vi "MCLB Test.vi"() -> ()   [LabVIEW 2013]
uses:
  <vilib>/NI/Tag Bus/tag/Data Type.ctl
  Table Manager/object ref.ctl
  <vilib>/NI/Tag Bus Data Framework/Configuration Editor/Classes/Engine Parent/Engine Parent Editor Node.lvclass
  <vilib>/NI/Tag Bus Data Framework/Configuration Editor/Classes/Module editor node/module editor node.lvclass
  Table Manager/references.ctl
  <vilib>/NI/Configuration Framework/Node/StopEvent.ctl
  <vilib>/NI/Configuration Framework/Node/RefreshUIEvent.ctl
  <vilib>/NI/Configuration Framework/Node/CacheState.ctl
  <vilib>/NI/Configuration Framework/Node/NodeChangeEvent.ctl
  <vilib>/NI/Configuration Framework/Node/NodeRef.ctl
  <vilib>/NI/Configuration Framework/Node/NISE_CEF_Node.lvclass
  <vilib>/NI/Tag Bus Data Framework/control module/editor node/channel action event.ctl
  <vilib>/NI/Tag Bus Data Framework/control module/editor node/dialog output action.ctl
  <vilib>/NI/Tag Bus Module Framework/channel/TBM channel.lvclass
  <vilib>/NI/Tag Bus/tag/tag descriptor.lvclass
  <vilib>/NI/AMC/Message Queue.ctl
  <vilib>/NI/AMC/Message.ctl
  <vilib>/NI/Tools/Keyed Array/KeyedArray.ctl
  <vilib>/NI/Configuration Framework/Node/UserEventRef.ctl
  <vilib>/NI/Configuration Framework/Controls/EventCluster.ctl
  Listbox/Multi Column Listbox.lvclass
  Listbox/Multi Column Listbox.lvclass/Multi Column Listbox.ctl
  Table Manager/Table Manager.lvclass/Table Manager.ctl
  Listbox/Write Listbox.vi
  Table Manager/Write Top VI.vi
  editor node/Table Test Editor Node.lvclass
  Table Manager/Table Manager.lvclass
  <vilib>/NI/Tag Bus Data Framework/control module/editor node/control module editor.lvclass
  <vilib>/NI/Tools/Keyed Array/Tools_KeyedArray.lvlib
  <vilib>/NI/AMC/AMC.lvlib
  <vilib>/NI/Configuration Framework/NISE_CEF_TreeControl.lvlib
panel:
  in  "References in":T1
  in  "object refs":T8
  in  "dt":T9
  in  "tag select":i32(listbox)=1
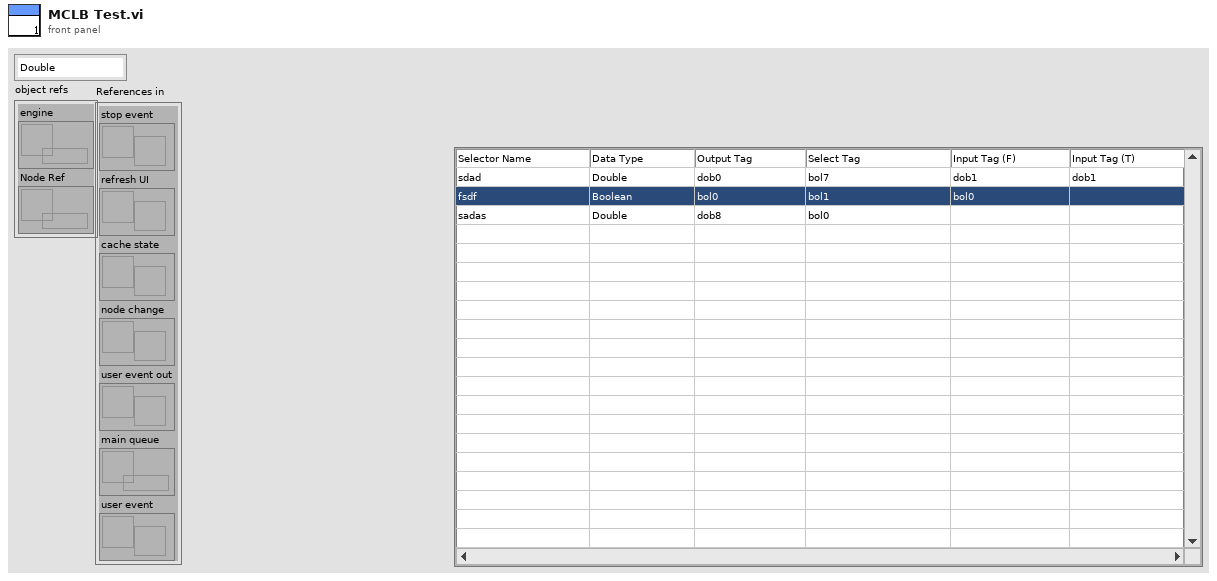
[diagram p1: front panel]
types:
  T1 = typedef "Table Manager.lvlib/Table Manager.lvclass/references.ctl" = cluster{"stop event":T2, "refresh UI":T3, "cache state":T4, "node change":T5, "user event out":refnum<user-event>, "main queue":T6, "user event":T7}
  T2 = typedef "NISE_CEF_Node.lvclass/StopEvent.ctl" = refnum<user-event>
  T3 = typedef "NISE_CEF_Node.lvclass/RefreshUIEvent.ctl" = refnum<user-event>
  T4 = typedef "NISE_CEF_Node.lvclass/CacheState.ctl" = refnum<user-event>
  T5 = typedef "NISE_CEF_Node.lvclass/NodeChangeEvent.ctl" = refnum<user-event>
  T6 = typedef "AMC.lvlib/Message Queue.ctl" = refnum<queue>
  T7 = typedef "NISE_CEF_Node.lvclass/UserEventRef.ctl" = refnum<user-event>
  T8 = typedef "Table Manager.lvlib/Table Manager.lvclass/object ref.ctl" = cluster{"engine":refnum<data-value>, "Node Ref":refnum<data-value>}
  T9 = typedef "tag bus.lvlib/tag descriptor.lvclass/Data Type.ctl" = enum16{"Double", "Single", "I64", "I32", "I16", "I8", "U64", "U32", "U16", "U8", "Boolean", "String", "Array of Double", "Array of Single", "Array of I64", "Array of I32", "Array of I16", "Array of I8", "Array of U64", "Array of U32", "Array of U16", "Array of U8", "Array of Boolean", "Array of String"}
  T10 = typedef "Table Manager.lvlib/Column.lvclass/Column Descriptor.ctl" = cluster{"name":string, "caption":string, "Column Type":T11, "Params":string, "AutoSizeMode":i32, "FillWeight":sgl, "MinWidth":u32, "tooltip":string, "Enum Reference":refnum<vi>, "Channel suffix":string, "Read Only":bool, "Call Back VI":T12, "DT Dependency":i32, "name dependency":i32, "data type":T9}
  T11 = typedef "Table Manager.lvlib/Column.lvclass/Column Type.ctl" = enum16{"String", "Mapping", "Channel Name", "Tag", "Enum", "Data Type", "Numeric"}
  T12 = typedef "Table Manager.lvlib/Table Manager.lvclass/Call Back Ref Type Def.ctl" = refnum<vi>
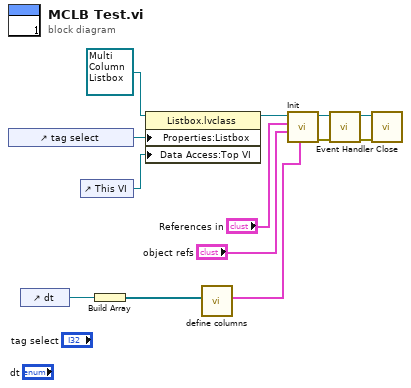
[diagram p0: block diagram]
diagram:
  n1 = control-ref of="tag select"() -> (w6:refnum<vi>)
  n2 = control-ref of="dt"() -> (w2:refnum<vi>)
  n3 = control-ref of="This VI"() -> (w5:refnum<vi>)
  n4 = Build Array(w2) -> (w1:refnum<vi>[])
  n5 = property class="Listbox.lvclass"(reference=refnum<class "Multi Column Listbox.lvclass"> refnum ("Table Manager.lvlib:Listbox.lvclass"), "Properties:Listbox"=w6, "Data Access:Top VI"=w5) -> (reference out=w3:refnum<class "Multi Column Listbox.lvclass">)  [unwired: 1 in, 1 out]
  n6 = call "define columns.vi"("Enum Array"=w1) -> ("Column Definition"=w7:T10[])  [unwired: 10 in]
  n7 = call-dynamic "Init.vi"("Column Definitions"=w7, "object refs"="object refs", "References in"="References in", "Multi Column Listbox in"=w3) -> ("error out"=w9:errorcluster, "Multi Column Listbox out"=w13:refnum<class "Multi Column Listbox.lvclass">)  [unwired: 5 in, 1 out]
  n8 = call-dynamic "Event Handler.vi"("error in"=w9, "Listbox in"=w13) -> ("error out"=w8:errorcluster, "Listbox out"=w12:refnum<class "Multi Column Listbox.lvclass">)  [unwired: 8 in]
  n9 = call-dynamic "Close.vi"("error in (no error)"=w8, "Multi Column Listbox in"=w12) -> ()  [unwired: 8 in, 2 out]
